vi "Write Data_Header_v2.vi"(10 "File path":path, 11 "Array":string[](array[string])) -> ()   [LabVIEW 2016]
uses:
  <vilib>/Utility/file.llb/Write To Spreadsheet File (string).vi
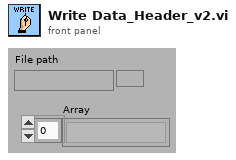
[diagram p1: front panel]
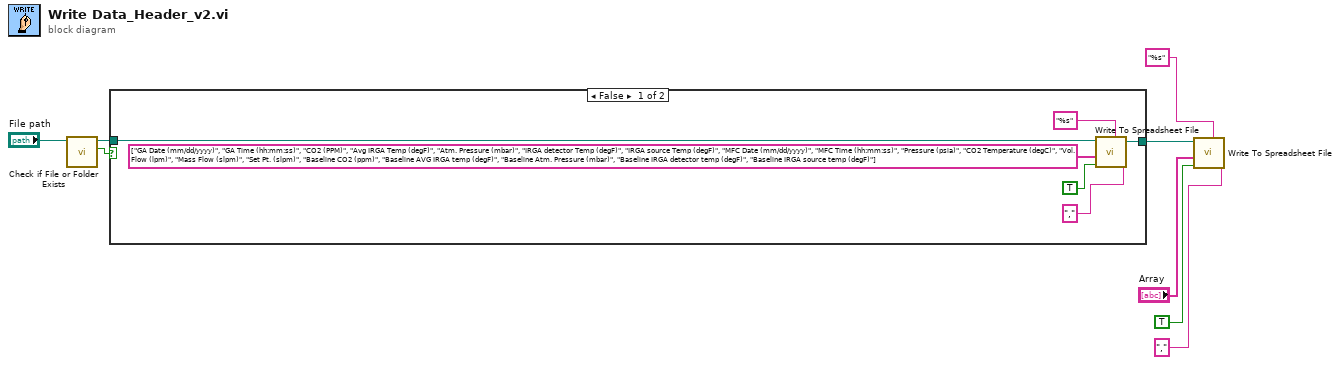
[diagram p0: block diagram]
diagram:
  n1 = call <vilib>:"Check if File or Folder Exists.vi"("path"="File path") -> ("file or folder exists?"=w8:bool, "dup path"=w7:path)  [unwired: 8 in, 1 out]
  n2 = case shown="False" w8 {
    tunnel: w7 -> [w11 w15]
    tunnel: [w9 w15] -> w2
    frame False {
      n3 = call-poly <vilib>:"Write To Spreadsheet File.vi"("delimiter (\\t)"="," ("delimiter (\\t)"), "format (%s)"="%s" ("format (%.3f)"), "append to file? (new file:F)"=TRUE, "1D data"=string[] ["GA Date (mm/dd/yyyy)", "GA Time (hh:mm:ss)", "CO2 (PPM)", "Avg IRGA Temp (degF)", "Atm. Pressure (mbar)", "IRGA detector Temp (degF)", "IRGA source Temp (degF)", "MFC Date (mm/dd/yyyy)", "MFC Time (hh:mm:ss)", "Pressure (psia)", "CO2 Temperature (degC)", "Vol. Flow (lpm)", "Mass Flow (slpm)", "Set Pt. (slpm)", "Baseline CO2 (ppm)", "Baseline AVG IRGA temp (degF)", "Baseline Atm. Pressure (mbar)", "Baseline IRGA detector temp (degF)", "Baseline IRGA source temp (degF)"], "file path (dialog if empty)"=w11) -> ("new file path (Not A Path if cancelled)"=w9:path)  [unwired: 3 in]
    }
    frame True {
    }
  }
  n4 = call-poly <vilib>:"Write To Spreadsheet File.vi"("delimiter (\\t)"="," ("delimiter (\\t)"), "format (%s)"="%s" ("format (%.3f)"), "append to file? (new file:F)"=TRUE, "1D data"="Array", "file path (dialog if empty)"=w2) -> ()  [unwired: 3 in, 1 out]
